vi "Recover One Persisted Value.vi"(8 "error in (no error)":errorcluster, 9 "Data Type":variant, 10 "Datum Name":string, 11 "Folder Path":path) -> (0 "error out":errorcluster, 2 "Recovered Value":T1)   [LabVIEW 2020, in "PersistToDiskTransport.lvclass"]
uses:
  PersistToDiskTransport.lvclass
  PersistToDiskTransport.lvclass/PersistToDiskTransport.ctl
  Recovered Value.ctl
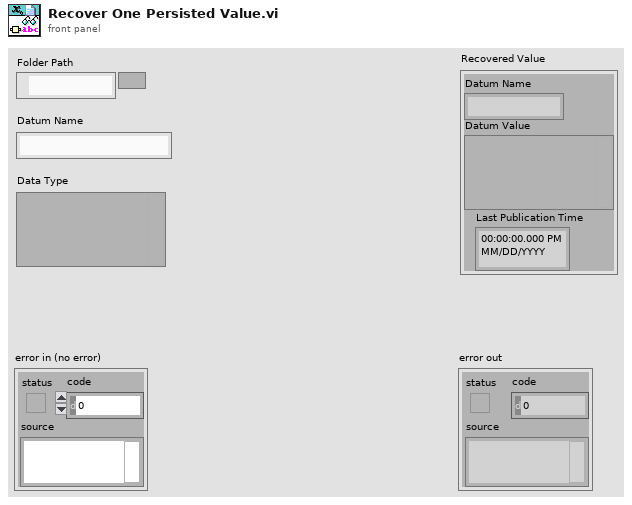
[diagram p1: front panel]
types:
  T1 = typedef "PersistToDiskTransport.lvclass/Recovered Value.ctl" = cluster{"Datum Name":string, "Datum Value":variant, "Last Publication Time":timestamp}
  T2 = cluster{"Datum Name":string, "type string":i16[], "data string":string, "Publication Time":timestamp}
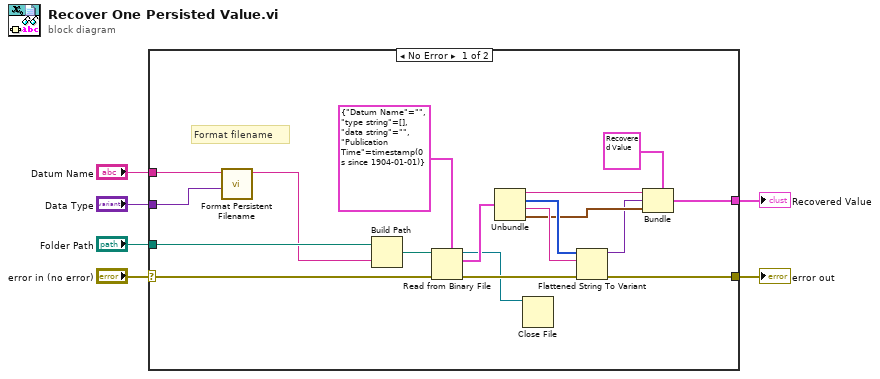
[diagram p0: block diagram]
diagram:
  n1 = case shown="No Error" "error in (no error)" {
    selector: "error in (no error)" -> [w23 w25]
    tunnel: [w21 w25] -> w5
    tunnel: "Folder Path" -> [w24 _]
    tunnel: [w19 _] -> w3
    tunnel: "Datum Name" -> [w9 _]
    tunnel: "Data Type" -> [w8 _]
    frame No Error {
      # "Format filename"
      n2 = call "Format Persistent Filename.vi"("Datum Type"=w8, "Datum Name"=w9) -> ("Filename"=w7:string)  [unwired: 9 in]
      n3 = Build Path(base path=w24, name or relative path=w7) -> (appended path=w18:path)
      n4 = Read from Binary File(5:T2 {"Datum Name"="", "type string"=[], "data string"="", "Publication Time"=timestamp(0 s since 1904-01-01)} ("cluster"), 8:w23, 11:w18) -> (0:w14:errorcluster, 2:w17:T2, 3:w10:refnum<file>)  [unwired: 3 in, 1 out]
      n5 = Unbundle(w17) -> ("Datum Name"=w13:string, "type string"=w16:i16[], "data string"=w15:string, "Publication Time"=w12:timestamp)
      n6 = Close File(refnum=w10) -> ()  [unwired: 1 in, 2 out]
      n7 = Flattened String To Variant(4:w14, 6:w15, 7:w16) -> (0:w21:errorcluster, 3:w11:variant)
      n8 = Bundle(cluster=T1 {"Datum Name"="", "Datum Value"=variant, "Last Publication Time"=timestamp(0 s since 1904-01-01)}, "Datum Name"=w13, "Datum Value"=w11, "Last Publication Time"=w12) -> (w19:T1)
    }
    frame Error {
    }
  }
  "error out" <- w5
  "Recovered Value" <- w3
